vi "Get Gyro at Time.vi"(8 "error in":errorcluster, 11 "Get ms ago":u32) -> (0 "error out":errorcluster, 3 "Angle":dbl)   [LabVIEW 2016, in "Path Track.lvlib"]
uses:
  Path Track.lvlib
  FGV Control.ctl
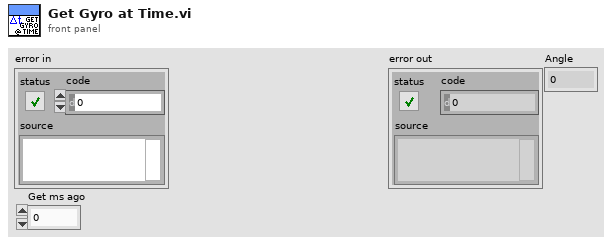
[diagram p1: front panel]
types:
  T1 = typedef "Path Track.lvlib/FGV Control.ctl" = enum16{"Allocate", "Get", "Append"}
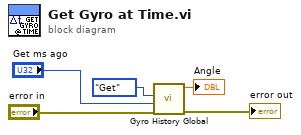
[diagram p0: block diagram]
diagram:
  n1 = call "Gyro History Global.vi"("error in"="error in", "Get ms ago"="Get ms ago", "Operation"=FGV_Control."Get") -> ("error out"=→"error out":errorcluster, "Angle"=→"Angle":dbl)  [unwired: 7 in]
